vi "ATF-CS-Log Analog Queues.vi"(8 "error in":errorcluster, 9 "Analog queues":refnum<queue>[](array[refnum]), 10 "Channel names":T1, 11 "tdms file in":refnum<k34>) -> (0 "error out":errorcluster, 3 "tdms ref out":refnum<k34>)   [LabVIEW 2022 SP3]
uses:
  <vilib>/Waveform/WDTOps.llb/WDT Get Waveform Time Array DBL.vi
panel:
  out "x":u32
  out "Waveform":waveform(dbl)[](array[waveform])
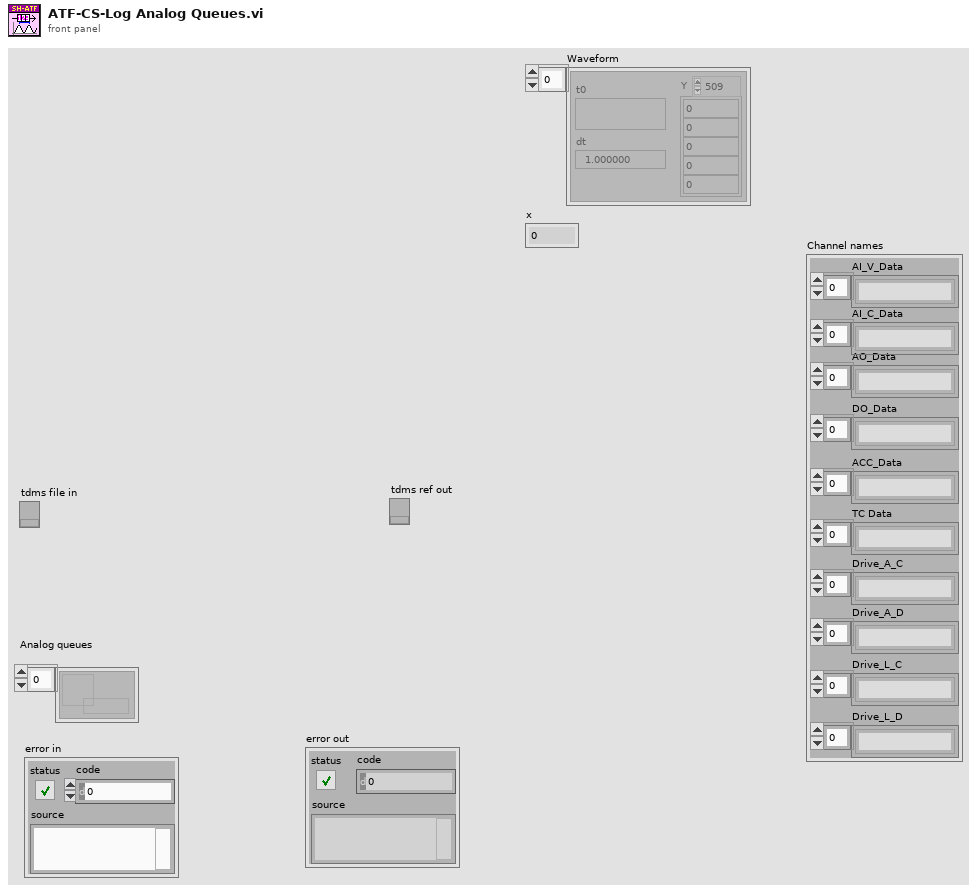
[diagram p1: front panel]
types:
  T1 = cluster{"AI_C_Data":string[], "AI_V_Data":string[], "AO_Data":string[], "DO_Data":string[], "ACC_Data":string[], "TC Data":string[], "Drive_A_C":string[], "Drive_A_D":string[], "Drive_L_C":string[], "Drive_L_D":string[]}
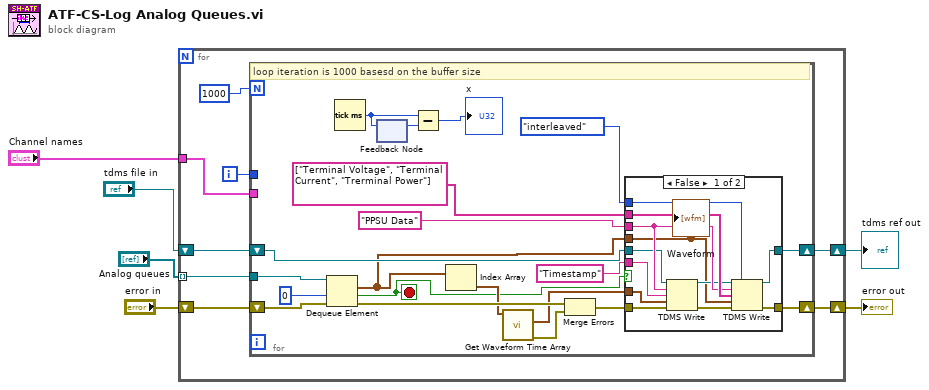
[diagram p0: block diagram]
diagram:
  n1 = for {
    tunnel: "Analog queues" -> [w13] mode=indexing
    shift-right: [w11] -> w4
    shift-left: "tdms file in" -> [w14]
    shift-right: [w9] -> w3
    shift-left: "error in" -> [w10]
    tunnel: "Channel names" -> [w7]
    i -> [w8]
    n2 = for {
      N: 1000 -> [_]
      tunnel: w13 -> [w31]
      shift-right: [w22] -> w11
      shift-left: w14 -> [w23]
      shift-right: [w27] -> w9
      shift-left: w10 -> [w30]
      tunnel: w8 -> [_]
      tunnel: w7 -> [_]
      stop <- w20 stop-if-true
      # "loop iteration is 1000 basesd on the buffer size"
      n3 = Dequeue Element(queue=w31, timeout in ms (-1)=0, error in (no error)=w30) -> (element=w19:waveform(dbl)[], timed out?=w20:bool, error out=w33:errorcluster)  [unwired: 1 out]
      n4 = Tick Count (ms)() -> (millisecond timer value=w17:u32)
      n5 = feedback #1() -> (w18:u32)  [unwired: 1 in]
      n6 = feedback-in #1(w17) -> ()
      n7 = Subtract(x=w17, y=w18) -> (x-y=→"x":u32)
      n8 = Index Array(array=w19) -> (element=w29:waveform(dbl))  [unwired: 1 in]
      n9 = call-poly <vilib>:"Get Waveform Time Array.vi"("waveform in"=w29) -> ("error out"=w32:errorcluster, "X array"=w24:timestamp[])  [unwired: 9 in]
      n10 = Merge Errors(w33, w32) -> (w28:errorcluster)
      n11 = case shown="False" w20 {
        tunnel: w28 -> [w46 w48]
        tunnel: [w44 w48] -> w27
        tunnel: string[] ["Terminal Voltage", "Terminal Current", "Trerminal Power"] -> [w43 _]
        tunnel: "PPSU Data" ("group name in (Untitled)") -> [w42 _]
        tunnel: "Timestamp" -> [w41 _]
        tunnel: w24 -> [w40 _]
        tunnel: w23 -> [w39 w47]
        tunnel: [w37 w47] -> w22
        tunnel: w19 -> [w36 _]
        tunnel: enum16{"decimated", "interleaved"}."interleaved" ("data layout (0:decimated)") -> [w35 _]
        frame False {
          n12 = TDMS Write(0:w39, 5:w42, 7:w41, 9:w40, 11:w46) -> (4:w38:refnum<k34>, 15:w45:errorcluster)  [unwired: 1 in, 2 out]
          n13 = TDMS Write(0:w38, 1:w35, 5:w42, 7:w43, 9:w36, 11:w45) -> (4:w37:refnum<k34>, 15:w44:errorcluster)  [unwired: 2 out]
          "Waveform" <- w36
        }
        frame True {
        }
      }
    }
  }
  "tdms ref out" <- w4
  "error out" <- w3
